vi "channel qualification test.vi"() -> ()   [LabVIEW 2013, in "CVT tests.lvlib"]
uses:
  CVT tests.lvlib
  <vilib>/NI/Tag Bus Module Framework/channel/channel classification.ctl
  configuration/CVT configuration.lvclass
  <vilib>/NI/Configuration Framework/serializable configuration/NISE_CEF_serializable configuration.lvclass/NISE_CEF_serializable configuration.ctl
  <vilib>/NI/Configuration Framework/serializable configuration/NISE_CEF_serializable configuration.lvclass
  <vilib>/NI/Tag Bus/tag/tag descriptor.lvclass/tag descriptor.ctl
  configuration/CVT configuration.lvclass/CVT configuration.ctl
  <vilib>/NI/Configuration Framework/serializable configuration/Read UID.vi
  configuration/Write channels.vi
  <vilib>/NI/Tag Bus Module Framework/channel/TBM channel.lvclass
  <vilib>/NI/Tag Bus/tag/tag descriptor.lvclass
  <vilib>/NI/Tag Bus Module Framework/module configuration/TBM module configuration.lvclass
  <vilib>/NI/LV Tools Palette/Misc/NISE Tools General.lvlib
panel:
  out "qualified channels OK":bool
  out "no err":errorcluster
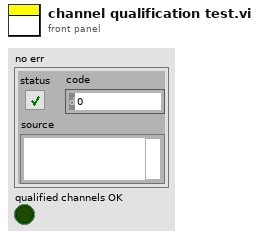
[diagram p1: front panel]
types:
  T1 = typedef "TBM channel.lvclass/channel classification.ctl" = enum16{"input data", "output data", "processing parameter", "processing result"}
  T2 = typedef "tag bus.lvlib/tag descriptor.lvclass/Data Type.ctl" = enum16{"Double", "Single", "I64", "I32", "I16", "I8", "U64", "U32", "U16", "U8", "Boolean", "String", "Array of Double", "Array of Single", "Array of I64", "Array of I32", "Array of I16", "Array of I8", "Array of U64", "Array of U32", "Array of U16", "Array of U8", "Array of Boolean", "Array of String"}
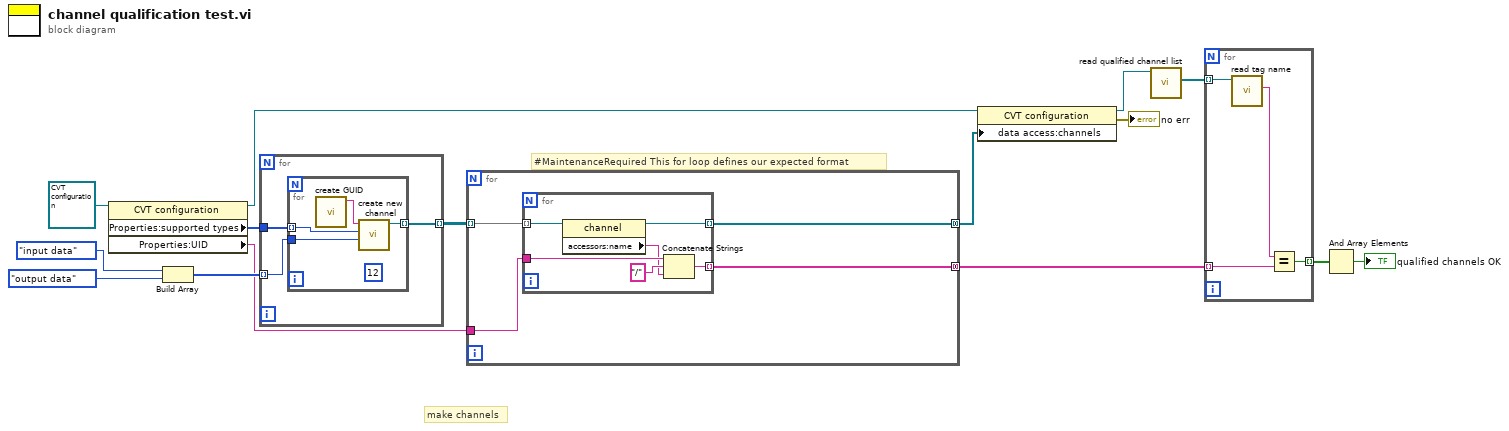
[diagram p0: block diagram]
diagram:
  # "#MaintenanceRequired This for loop defines our expected format"
  # "make channels"
  n1 = property class="CVT configuration"(reference=refnum<class "CVT configuration.lvclass"> refnum ("tag bus configurable plugin module configuration")) -> (reference out=w12:refnum<class "CVT configuration.lvclass">, "Properties:supported types"=w11:T2[], "Properties:UID"=w1:string)  [unwired: 1 in, 1 out]
  n2 = Build Array(channel_classification."input data" ("channel classification"), channel_classification."output data" ("channel classification")) -> (w13:T1[])
  n3 = for {
    tunnel: w13 -> [w18] mode=indexing
    tunnel: [w16] -> w10 mode=indexing
    tunnel: w11 -> [w17]
    n4 = for {
      tunnel: w18 -> [w21]
      tunnel: [w22] -> w16 mode=indexing
      tunnel: w17 -> [w20] mode=indexing
      (unwired) 12
      n5 = call <vilib>:"create GUID.vi"() -> ("UUID"=w19:string)  [unwired: 11 in]
      n6 = call <vilib>:"create new channel.vi"("channel classification"=w21, "data type"=w20, "channel name"=w19) -> ("channel"=w22:refnum<class "TBM channel.lvclass">)  [unwired: 8 in]
    }
  }
  n7 = for {
    tunnel: [w26] -> w2 mode=concatenating
    tunnel: w10 -> [w25] mode=indexing
    tunnel: w1 -> [w24]
    tunnel: [w23] -> w6 mode=concatenating
    n8 = for {
      tunnel: [w27] -> w26 mode=indexing
      tunnel: w25 -> [w32] mode=indexing
      tunnel: w24 -> [w31]
      tunnel: [w28] -> w23 mode=indexing
      n9 = property class="channel"(reference=w32) -> (reference out=w27:refnum<class "TBM channel.lvclass">, "accessors:name"=w29:string)  [unwired: 1 in, 1 out]
      n10 = Concatenate Strings(w31, "/" ("string"), w29) -> (w28:string)
    }
  }
  n11 = property class="CVT configuration"(reference=w12, "data access:channels"=w2) -> (reference out=w3:refnum<class "CVT configuration.lvclass">, error out=→"no err":errorcluster)  [unwired: 1 in]
  n12 = call <vilib>:"read qualified channel list.vi"("module configuration in"=w3) -> ("qualified channels"=w7:refnum<class "TBM channel.lvclass">[])  [unwired: 9 in, 1 out]
  n13 = for {
    tunnel: w6 -> [w35] mode=indexing
    tunnel: w7 -> [w36] mode=indexing
    tunnel: [w33] -> w9 mode=indexing
    n14 = call <vilib>:"read tag name.vi"("system tag in"=w36) -> ("name"=w34:string)  [unwired: 8 in, 2 out]
    n15 = Equal?(x=w34, y=w35) -> (x = y?=w33:bool)
  }
  n16 = And Array Elements(Boolean array=w9) -> (logical AND=→"qualified channels OK":bool)
